vi "[Global] Analyze Image.vi"() -> ()   [LabVIEW 2019]
panel:
  out "Analyze Image":T1(plugin-control)
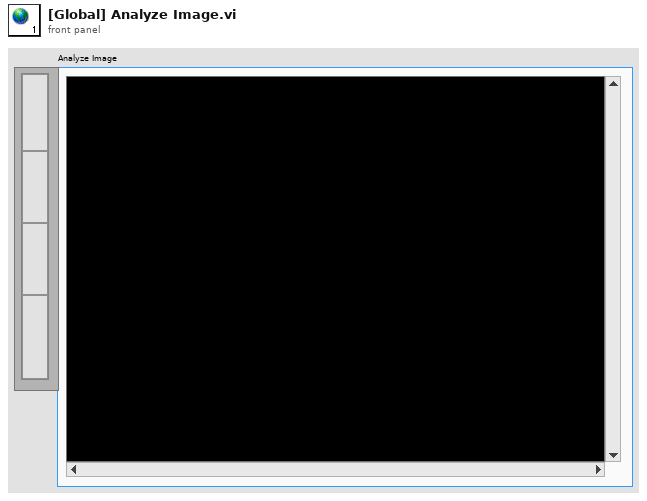
[diagram p1: front panel]
types:
  T1 = typedef "IMAQ Image.ctl" = refnum<image>
diagram:
